vi "Configure.vi"(8 "error in (no error)":errorcluster, 11 "Cascade in":refnum<class "Cascade.lvclass">) -> (0 "error out":errorcluster, 2 "cancelled?":bool, 3 "Cascade out":refnum<class "Cascade.lvclass">)   [LabVIEW 2012, in "Cascade.lvclass"]
doc: "The configure method configures the details for the RabbitMQ connection, the observers and the mapping script.\n\nIn the derived class, make a call to the parent for setting these parameters."
uses:
  Cascade.lvclass
  <vilib>/Distrio/Murmex/Murmex/Murmex.lvclass
  <vilib>/Utility/miscctls.llb/LVPointTypeDef.ctl
  timing mode.ctl
  Trigger edge.ctl
panel:
  in  "Tab Control":enum32{"camera", "debug"}(tab)
  in  "Trigger Edge":T1 items=["Leading edge"=1, "Falling edge"=2]
  in  "Timing mode":T2 items=["Free run"=1, "External trigger"=2, "Strobe mode  (ext trigger)"=3, "Bulb mode (ext trigger)"=4, "Variable mode (ext trigger)"=5, "Flash mdoe (ext trigger)"=6]
  in  "button:call parent":bool
  in  "button:ok":bool
  in  "button:cancel":bool
  # "RabbitMQ parameters"
  # "Window position"
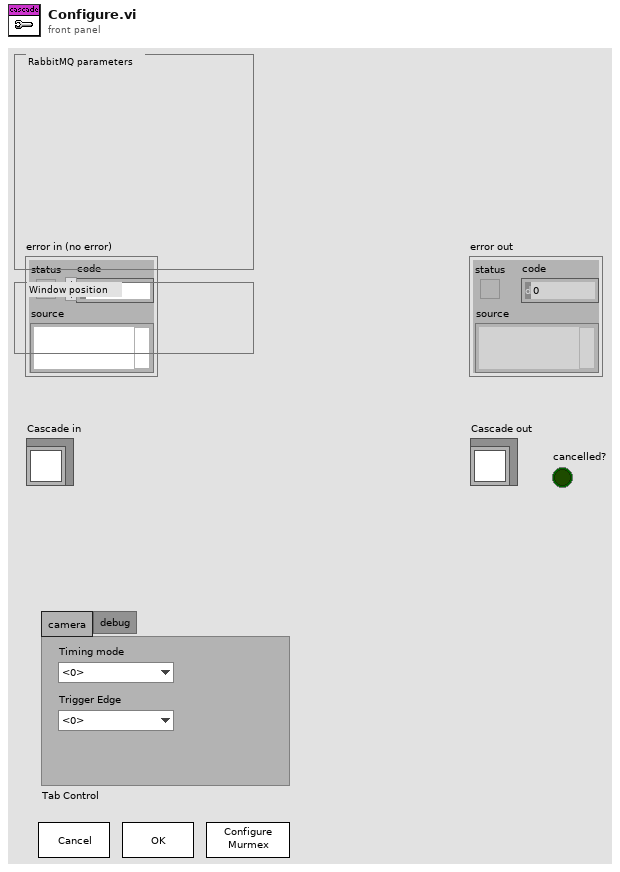
[diagram p1: front panel]
types:
  T1 = typedef "Cascade.lvclass/Trigger edge.ctl" = u32
  T2 = typedef "Cascade.lvclass/timing mode.ctl" = u32
  T3 = typedef "LVPointTypeDef.ctl" = cluster{"Horizontal":i16, "Vertical":i16}
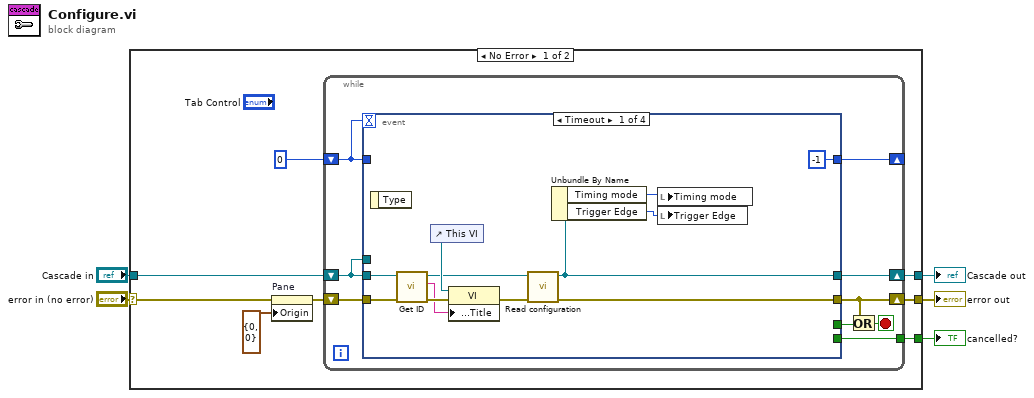
[diagram p0: block diagram]
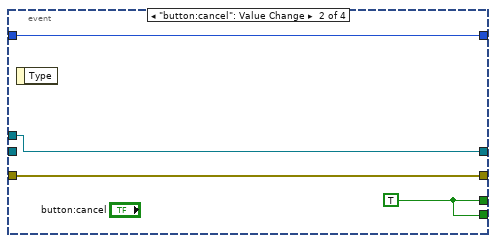
[diagram p2: hidden frame]
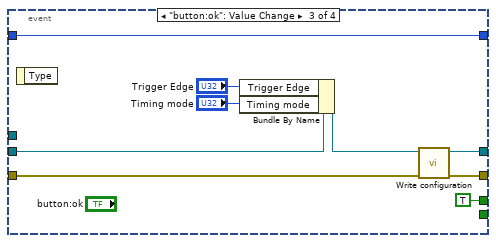
[diagram p3: hidden frame]
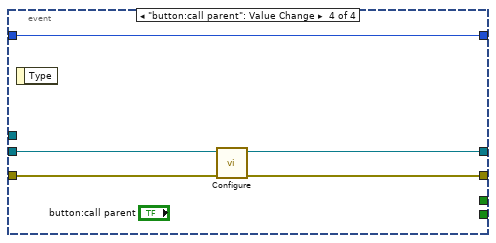
[diagram p4: hidden frame]
diagram:
  n1 = case shown="No Error" "error in (no error)" {
    selector: "error in (no error)" -> [w12 w53]
    tunnel: "Cascade in" -> [w9 w54]
    tunnel: [w10 w53] -> w3
    tunnel: [w7 w54] -> w2
    tunnel: [w6 _] -> w1
    frame No Error {
      n2 = property on="Pane" class="Pane"(error in=w12, "Origin"=T3 {"Horizontal"=0, "Vertical"=0}) -> (error out=w11:errorcluster)  [unwired: 1 in, 1 out]
      n3 = while {
        shift-right: [w17] -> w10
        shift-left: w11 -> [w22]
        shift-right: [w18] -> w7
        shift-left: w9 -> [w21]
        shift-right: [w19] -> _
        shift-left: 0 -> [w20]
        tunnel: [w14] -> w6
        stop <- w16 stop-if-true
        n4 = event shown="[0] Timeout" {
          selector: _ -> [_ _ _ _]
          dyn-events: _ -> [_ _ _ _]
          timeout: w20 -> [_ _ _ _]
          tunnel: w22 -> [w33 w37 w44 w52]
          tunnel: w21 -> [w32 _ w42 w50]
          tunnel: w21 -> [_ w38 _ _]
          tunnel: w20 -> [_ w35 w47 w48]
          tunnel: [-1 w35 w47 w48] -> w19
          tunnel: [w26 w38 w45 w49] -> w18
          tunnel: [w25 w37 w46 w51] -> w17
          tunnel: [_ w36 TRUE ("cancelled?") _] -> w15
          tunnel: [_ w36 _ _] -> w14
          event Timeout {
            n5 = event-data() -> ()  [unwired: 1 in, 1 out]
            n6 = call <vilib>:"Get ID.vi"("error in (no error)"=w33, "Murmex in"=w32) -> ("error out"=w31:errorcluster, "component id"=w27:string, "Murmex out"=w28:refnum<class "Cascade.lvclass">)  [unwired: 7 in]
            n7 = control-ref of="This VI"() -> (w30:refnum<vi>)
            n8 = property class="VI"(reference=w30, error in=w31, "Front Panel.Title"=w27) -> (error out=w29:errorcluster)  [unwired: 1 out]
            n9 = call <vilib>:"Read configuration.vi"("error in (no error)"=w29, "Murmex in"=w28) -> ("error out"=w25:errorcluster, "Murmex out"=w26:refnum<class "Cascade.lvclass">)  [unwired: 7 in, 1 out]
            n10 = Unbundle By Name(w26) -> ("Timing mode"=w24:T2, "Trigger Edge"=w23:T1)
            n11 = local write "Timing mode"(w24) -> ()
            n12 = local write "Trigger Edge"(w23) -> ()
          }
          event "button:cancel": Value Change {
            w36 = TRUE ("cancelled?")
            n13 = event-data() -> ()  [unwired: 1 in, 1 out]
          }
          event "button:ok": Value Change {
            n14 = event-data() -> ()  [unwired: 1 in, 1 out]
            n15 = Bundle By Name(cluster=w42, "Trigger Edge"="Trigger Edge", "Timing mode"="Timing mode") -> (w43:refnum<class "Cascade.lvclass">)
            n16 = call <vilib>:"Write configuration.vi"("error in (no error)"=w44, "Murmex in"=w43) -> ("error out"=w46:errorcluster, "Murmex out"=w45:refnum<class "Cascade.lvclass">)  [unwired: 8 in]
          }
          event "button:call parent": Value Change {
            n17 = event-data() -> ()  [unwired: 1 in, 1 out]
            n18 = call-parent "Configure.vi"("error in (no error)"=w52, "Murmex in"=w50) -> ("error out"=w51:errorcluster, "Murmex out"=w49:refnum<class "Cascade.lvclass">)  [unwired: 7 in, 1 out]
          }
        }
        n19 = Or(x=w17, y=w15) -> (x .or. y?=w16:bool)
      }
    }
    frame Error {
    }
  }
  "error out" <- w3
  "Cascade out" <- w2
  "cancelled?" <- w1
